vi "ConnectCheck.vi"   [LabVIEW 2018]
types:
  T1 = cluster{"Selected Index []":i32[], "Selected Items":string[]}
  T2 = enum16{"功率测量", "能量测量", "光谱测量", "时间波形", "偏振测量", "近远场"}
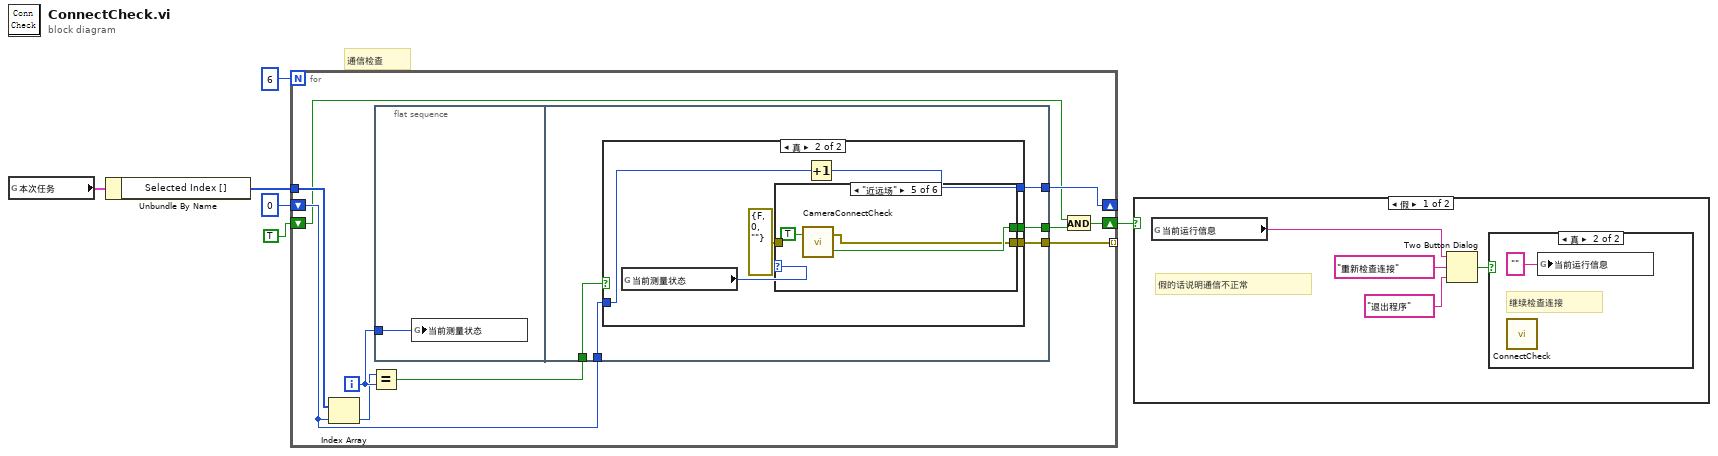
[diagram p0: block diagram]
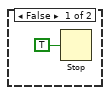
[diagram p2: hidden frame]
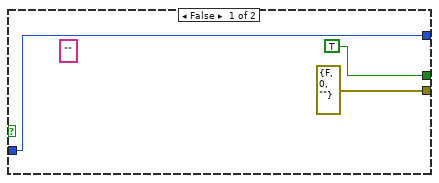
[diagram p4: hidden frame]
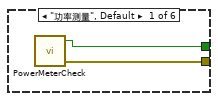
[diagram p5: hidden frame]
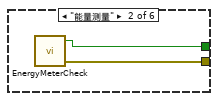
[diagram p6: hidden frame]
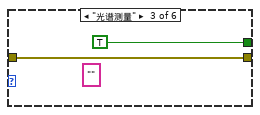
[diagram p7: hidden frame]
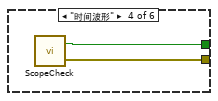
[diagram p8: hidden frame]
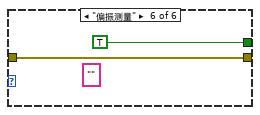
[diagram p9: hidden frame]
diagram:
  # "通信检查"
  n1 = global read "参数.vi" "本次任务"() -> (w4:T1)
  n2 = Unbundle By Name(w4) -> ("Selected Index []"=w3:i32[])
  n3 = for {
    N: 6 -> [_]
    tunnel: w3 -> [w16]
    shift-right: [w12] -> _
    shift-left: 0 -> [w11]
    shift-right: [w8] -> w1
    shift-left: TRUE -> [w9]
    tunnel: [w7] -> _ mode=indexing
    i -> [w15]
    n4 = Index Array(array=w16, index=w11) -> (element=w13:i32)
    n5 = Equal?(x=w13, y=w15) -> (x = y?=w14:bool)
    n6 = flat-sequence {
      tunnel: w15 -> [w17]
      tunnel: w14 -> [w22]
      tunnel: w11 -> [w20]
      tunnel: [w21] -> w12
      tunnel: [w19] -> w10
      tunnel: [w18] -> w7
      frame #0 {
        n7 = global write "参数.vi" "当前测量状态"(w17) -> ()
      }
      frame #1 {
        n8 = case shown="真" w22 {
          tunnel: w20 -> [w25 w28]
          tunnel: [w25 w31] -> w21
          tunnel: [TRUE ("通信正常？") w27] -> w19
          tunnel: [errorcluster {"status"=FALSE, "code"=0, "source"=""} ("error out") w26] -> w18
          frame False {
            (unwired) ""
          }
          frame True {
            n9 = global read "参数.vi" "当前测量状态"() -> (w30:T2)
            n10 = case shown="\"近远场\"" w30 {
              tunnel: errorcluster {"status"=FALSE, "code"=0, "source"=""} ("error out") -> [_ _ w36 _ _ w43]
              tunnel: [w33 w35 TRUE w39 w42 TRUE] -> w27
              tunnel: [w32 w34 w36 w38 w41 w43] -> w26
              frame "功率测量", Default {
                n11 = call "PowerMeterCheck.vi"() -> ("通信正常？"=w33:bool, "错误输出"=w32:errorcluster)  [unwired: 3 in]
              }
              frame "能量测量" {
                n12 = call "EnergyMeterCheck.vi"() -> ("通信正常？"=w35:bool, "错误输出"=w34:errorcluster)  [unwired: 3 in]
              }
              frame "光谱测量" {
                (unwired) "" ("任务")
              }
              frame "时间波形" {
                n13 = call "ScopeCheck.vi"() -> ("错误输出"=w38:errorcluster, "通信正常？"=w39:bool)  [unwired: 2 in]
              }
              frame "近远场" {
                n14 = call "CameraConnectCheck.vi"("是否通信检查"=TRUE) -> ("通信正常？"=w42:bool, "error out"=w41:errorcluster)  [unwired: 1 in]
              }
              frame "偏振测量" {
                (unwired) "" ("任务")
              }
            }
            n15 = Increment(x=w28) -> (x+1=w31:i32)
          }
        }
      }
    }
    n16 = And(x=w9, y=w10) -> (x .and. y?=w8:bool)
  }
  n17 = case shown="假" w1 {
    frame False {
      # "假的话说明通信不正常"
      n18 = global read "globalMessage.vi" "当前运行信息"() -> (w45:string)
      n19 = Two Button Dialog(message=w45, 1:"退出程序" ("F按钮名称（“取消”）"), 2:"重新检查连接" ("T按钮名称（“确定”）")) -> (T button?=w46:bool)
      n20 = case shown="真" w46 {
        frame False {
          n21 = Stop(stop? (T)=TRUE) -> ()
        }
        frame True {
          # "继续检查连接"
          n22 = call "ConnectCheck.vi"() -> ()  [unwired: 12 in]
          n23 = global write "globalMessage.vi" "当前运行信息"("" ("当前运行信息")) -> ()
        }
      }
    }
    frame True {
    }
  }
